vi "write connection list to top file.vi"(8 "error in (no error)":errorcluster, 10 "ConnectionList":T2[](array[typedef]), 11 "Refnum in":T1) -> (0 "error out":errorcluster, 3 "Refnum out":T1)   [LabVIEW 2015, in "SLSC Switch.lvlib" / "SLSC Switch.lvclass"]
uses:
  SLSC Switch.lvclass
  Controls/JSON.ConnectionList.ctl
  <vilib>/Utility/config.llb/Config Data RefNum.ctl
  <vilib>/Utility/config.llb/Write Key (String).vi
  <vilib>/Utility/config.llb/NI_LVConfig.lvlib
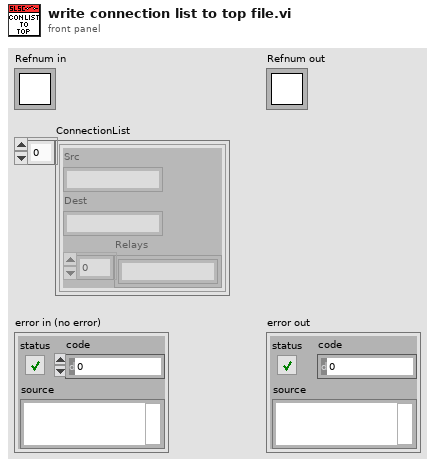
[diagram p1: front panel]
types:
  T1 = typedef "NI_LVConfig.lvlib/Config Data RefNum.ctl" = refnum<k1>
  T2 = typedef "SLSC Switch.lvlib/SLSC Switch.lvclass/JSON.ConnectionList.ctl" = cluster{"Src":string, "Dest":string, "Relays":string[]}
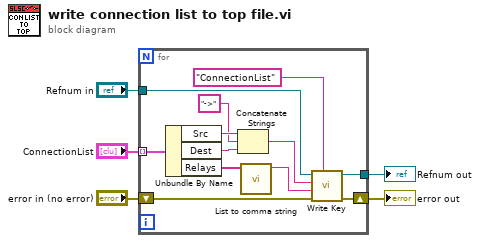
[diagram p0: block diagram]
diagram:
  n1 = for {
    tunnel: "Refnum in" -> [w9]
    shift-right: [w10] -> w5
    shift-left: "error in (no error)" -> [w11]
    tunnel: [w8] -> w2
    tunnel: "ConnectionList" -> [w6] mode=indexing
    n2 = Unbundle By Name(w6) -> ("Src"=w17:string, "Dest"=w15:string, "Relays"=w13:string[])
    n3 = Concatenate Strings(w17, "->" ("string"), w15) -> (w14:string)
    n4 = call "List to comma string.vi"("Array"=w13) -> ("String"=w12:string)  [unwired: 10 in]
    n5 = call-poly <vilib>:"Write Key.vi"("section"="ConnectionList", "error in (no error)"=w11, "value"=w12, "key"=w14, "refnum"=w9) -> ("error out"=w10:errorcluster, "refnum out"=w8:T1)  [unwired: 4 in, 1 out]
  }
  "error out" <- w5
  "Refnum out" <- w2
